vi "FT_Set_Baud_Rate.vi"(2 "Baud Rate":u32, 3 "Handle":u32) -> (0 "FT_Status":u32, 1 "Handle 2":u32)   [LabVIEW 2011]
uses:
  FTD2XX.dll
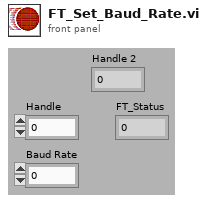
[diagram p1: front panel]
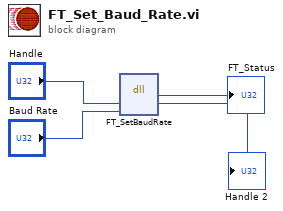
[diagram p0: block diagram]
diagram:
  n1 = dll-call lib="D:/WORK/LabView/#Avesta/D2XX_Functions_7.0/FTD2XX.dll" fn="FT_SetBaudRate"("Handle"="Handle", "BaudRate"="Baud Rate") -> ("FT_Status"=→"FT_Status":u32, "Handle"=→"Handle 2":u32)  [unwired: 4 in, 2 out]
